vi "niScope Query Vertical.vi"(0 "instrument handle":refnum<k15>, 5 "channel name":string="0", 11 "error in":errorcluster {"code" format="%.0x"}) -> (3 "probe attenuation":dbl=1.0 format="%.1f", 4 "instrument handle out":refnum<k15>, 6 "vertical range":dbl=10.0 format="%.2f", 8 "vertical coupling":T1=1 items=["AC", "DC", "Ground"], 10 "vertical offset":dbl format="%.4f", 13 "gain":dbl, 14 "channel enabled":bool=TRUE, 15 "error out":errorcluster {"code" format="%.0x"})   [LabVIEW 2011]
doc: "This VI configures the common properties of the oscilloscope's vertical subsystem for the specified channel."
uses:
  <instrlib>/niScope/Controls/niScope vertical coupling.ctl
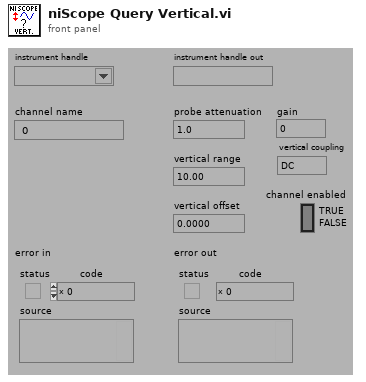
[diagram p1: front panel]
types:
  T1 = typedef "niScope vertical coupling.ctl" = i32
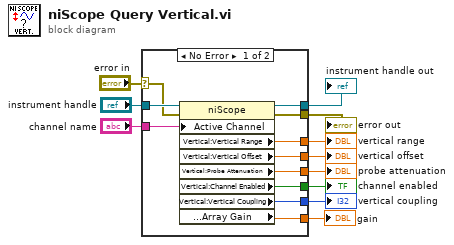
[diagram p0: block diagram]
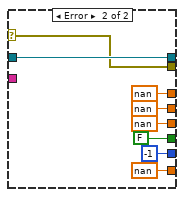
[diagram p2: hidden frame]
diagram:
  n1 = case shown="No Error" "error in" {
    selector: "error in" -> [w19 w29]
    tunnel: [w21 w29] -> w11
    tunnel: "instrument handle" -> [w22 w30]
    tunnel: [w20 w30] -> w9
    tunnel: "channel name" -> [w18 _]
    tunnel: [w17 nan ("Vertical Range")] -> w6
    tunnel: [w16 nan ("Vertical Offset")] -> w5
    tunnel: [w15 nan ("Probe Attenuation")] -> w4
    tunnel: [w14 FALSE ("Channel Enabled")] -> w3
    tunnel: [w13 -1 ("Vertical Coupling")] -> w2
    tunnel: [w12 nan ("Probe Attenuation")] -> w1
    frame No Error {
      n2 = property class="niScope"(reference=w22, error in=w19, "Active Channel"=w18) -> (reference out=w20:refnum<k15>, error out=w21:errorcluster, "Vertical:Vertical Range"=w17:dbl, "Vertical:Vertical Offset"=w16:dbl, "Vertical:Probe Attenuation"=w15:dbl, "Vertical:Channel Enabled"=w14:bool, "Vertical:Vertical Coupling"=w13:i32, "Waveform Measurement:Array Gain"=w12:dbl)
    }
    frame Error {
    }
  }
  "error out" <- w11
  "instrument handle out" <- w9
  "vertical range" <- w6
  "vertical offset" <- w5
  "vertical coupling" <- w2
  "probe attenuation" <- w4
  "channel enabled" <- w3
  "gain" <- w1
